vi "Get Guide_RA_DEC.vi"(8 "error in (no error)":errorcluster, 11 "S4GUI in":refnum<class "S4GUI.lvclass">) -> (0 "error out":errorcluster, 3 "S4GUI out":refnum<class "S4GUI.lvclass">)   [LabVIEW 2018, in "S4GUI.lvclass"]
uses:
  S4GUI.lvclass
  S4GUI.lvclass/S4GUI.ctl
  Acquisition/Acquisition.lvclass
  Channel/Channel.lvclass
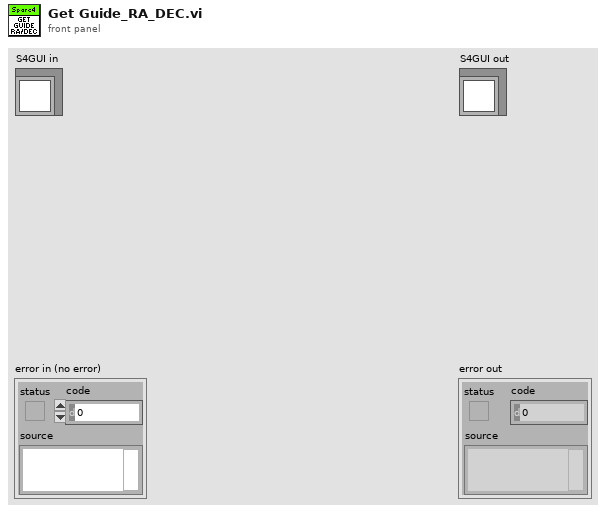
[diagram p1: front panel]
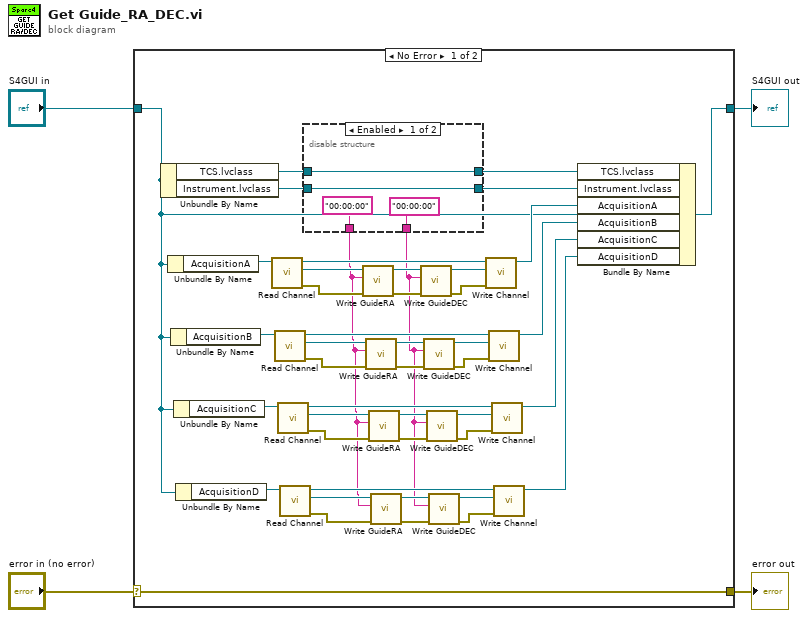
[diagram p0: block diagram]
diagram:
  n1 = case shown="No Error" "error in (no error)" {
    selector: "error in (no error)" -> [w49 w57]
    tunnel: [w49 w57] -> w3
    tunnel: [w36 w56] -> w1
    tunnel: "S4GUI in" -> [w10 w56]
    frame No Error {
      n2 = Unbundle By Name(w10) -> ("TCS.lvclass"=w48:refnum<class "TCS.lvclass">, "Instrument.lvclass"=w45:refnum<class "Instrument.lvclass">)
      n3 = Unbundle By Name(w10) -> ("AcquisitionA"=w44:refnum<class "Acquisition.lvclass">)
      n4 = Unbundle By Name(w10) -> ("AcquisitionB"=w34:refnum<class "Acquisition.lvclass">)
      n5 = Unbundle By Name(w10) -> ("AcquisitionC"=w26:refnum<class "Acquisition.lvclass">)
      n6 = Unbundle By Name(w10) -> ("AcquisitionD"=w18:refnum<class "Acquisition.lvclass">)
      n7 = call-dynamic "Read Channel.vi"("Acquisition in"=w44) -> ("error out"=w39:errorcluster, "Channel.lvclass"=w42:refnum<class "Channel.lvclass">, "Acquisition out"=w43:refnum<class "Acquisition.lvclass">)  [unwired: 8 in]
      n8 = call-dynamic "Read Channel.vi"("Acquisition in"=w34) -> ("error out"=w29:errorcluster, "Channel.lvclass"=w32:refnum<class "Channel.lvclass">, "Acquisition out"=w33:refnum<class "Acquisition.lvclass">)  [unwired: 8 in]
      n9 = call-dynamic "Read Channel.vi"("Acquisition in"=w26) -> ("error out"=w21:errorcluster, "Channel.lvclass"=w24:refnum<class "Channel.lvclass">, "Acquisition out"=w25:refnum<class "Acquisition.lvclass">)  [unwired: 8 in]
      n10 = call-dynamic "Read Channel.vi"("Acquisition in"=w18) -> ("error out"=w13:errorcluster, "Channel.lvclass"=w16:refnum<class "Channel.lvclass">, "Acquisition out"=w17:refnum<class "Acquisition.lvclass">)  [unwired: 8 in]
      n11 = disable-structure shown="Enabled" {
        disable-tunnel: ["00:00:00" _] -> w6
        disable-tunnel: [w52 w55] -> w47
        disable-tunnel: w48 -> [w52 w55]
        disable-tunnel: [w51 w54] -> w46
        disable-tunnel: w45 -> [w51 w54]
        disable-tunnel: ["00:00:00" _] -> w5
        frame Enabled {
        }
        frame Disabled {
          # "Calcula GuideRA e GuideDEC\na partir de RA, DEC e GMIR."
        }
      }
      n12 = call-dynamic "Write GuideRA.vi"("error in (no error)"=w39, "GuideRA"=w6, "Channel in"=w42) -> ("error out"=w38:errorcluster, "Channel out"=w41:refnum<class "Channel.lvclass">)  [unwired: 7 in]
      n13 = call-dynamic "Write GuideRA.vi"("error in (no error)"=w29, "GuideRA"=w6, "Channel in"=w32) -> ("error out"=w28:errorcluster, "Channel out"=w31:refnum<class "Channel.lvclass">)  [unwired: 7 in]
      n14 = call-dynamic "Write GuideRA.vi"("error in (no error)"=w21, "GuideRA"=w6, "Channel in"=w24) -> ("error out"=w20:errorcluster, "Channel out"=w23:refnum<class "Channel.lvclass">)  [unwired: 7 in]
      n15 = call-dynamic "Write GuideRA.vi"("error in (no error)"=w13, "GuideRA"=w6, "Channel in"=w16) -> ("error out"=w12:errorcluster, "Channel out"=w15:refnum<class "Channel.lvclass">)  [unwired: 7 in]
      n16 = call-dynamic "Write GuideDEC.vi"("error in (no error)"=w38, "GuideDEC"=w5, "Channel in"=w41) -> ("error out"=w37:errorcluster, "Channel out"=w40:refnum<class "Channel.lvclass">)  [unwired: 7 in]
      n17 = call-dynamic "Write GuideDEC.vi"("error in (no error)"=w28, "GuideDEC"=w5, "Channel in"=w31) -> ("error out"=w27:errorcluster, "Channel out"=w30:refnum<class "Channel.lvclass">)  [unwired: 7 in]
      n18 = call-dynamic "Write GuideDEC.vi"("error in (no error)"=w20, "GuideDEC"=w5, "Channel in"=w23) -> ("error out"=w19:errorcluster, "Channel out"=w22:refnum<class "Channel.lvclass">)  [unwired: 7 in]
      n19 = call-dynamic "Write GuideDEC.vi"("error in (no error)"=w12, "GuideDEC"=w5, "Channel in"=w15) -> ("error out"=w11:errorcluster, "Channel out"=w14:refnum<class "Channel.lvclass">)  [unwired: 7 in]
      n20 = call-dynamic "Write Channel.vi"("error in (no error)"=w37, "Channel.lvclass"=w40, "Acquisition in"=w43) -> ("Acquisition out"=w35:refnum<class "Acquisition.lvclass">)  [unwired: 7 in, 1 out]
      n21 = call-dynamic "Write Channel.vi"("error in (no error)"=w27, "Channel.lvclass"=w30, "Acquisition in"=w33) -> ("Acquisition out"=w9:refnum<class "Acquisition.lvclass">)  [unwired: 7 in, 1 out]
      n22 = call-dynamic "Write Channel.vi"("error in (no error)"=w19, "Channel.lvclass"=w22, "Acquisition in"=w25) -> ("Acquisition out"=w8:refnum<class "Acquisition.lvclass">)  [unwired: 7 in, 1 out]
      n23 = call-dynamic "Write Channel.vi"("error in (no error)"=w11, "Channel.lvclass"=w14, "Acquisition in"=w17) -> ("Acquisition out"=w7:refnum<class "Acquisition.lvclass">)  [unwired: 7 in, 1 out]
      n24 = Bundle By Name(cluster=w10, "TCS.lvclass"=w47, "Instrument.lvclass"=w46, "AcquisitionA"=w35, "AcquisitionB"=w9, "AcquisitionC"=w8, "AcquisitionD"=w7) -> (w36:refnum<class "S4GUI.lvclass">)
    }
    frame Error {
    }
  }
  "error out" <- w3
  "S4GUI out" <- w1
